vi "programacion practica de examen1.vi"() -> ()   [LabVIEW 2011]
panel:
  out "Array":T1(array[cluster]) {"diesel" scale=0.0..500.0; "Gasolina r" scale=0.0..500.0; "Gasolina S" scale=0.0..500.0}
  # "Existen 5 estaciones de servicio, ud debera de guardar las\nmediciones de los tanques de combustible de cada una de las\nestaciones de servicio y obtener el promedio mayor y menor\npor cada una de las estaciones y luego guardar los datos \nen un archivo de texto."
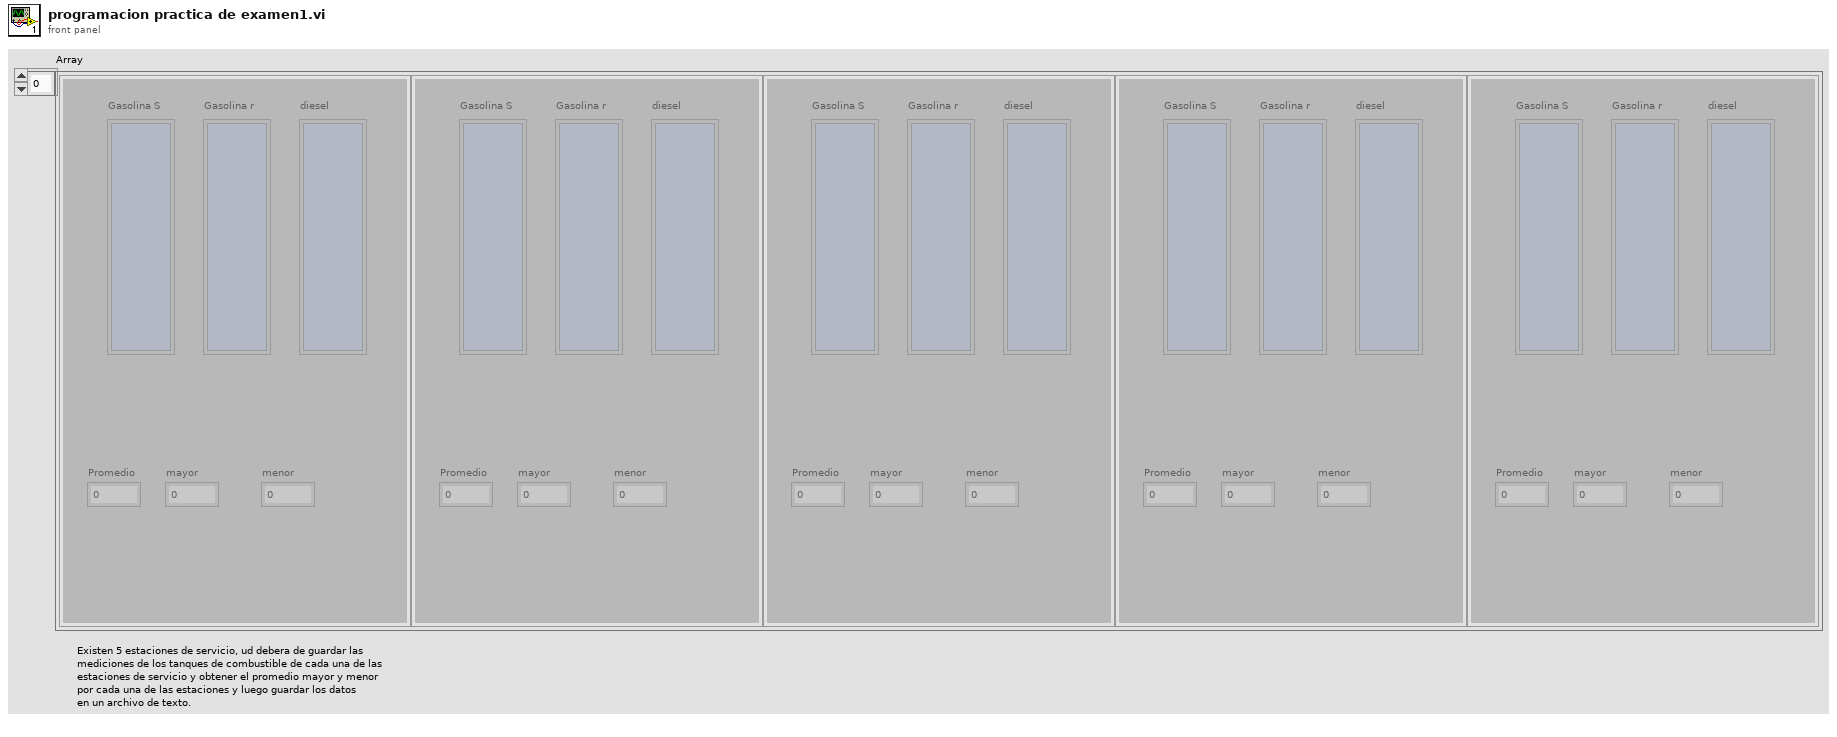
[diagram p1: front panel]
types:
  T1 = cluster{"Gasolina S":i32, "Gasolina r":i32, "diesel":i32, "Promedio":dbl, "mayor":dbl, "menor":dbl}[]
  T2 = enum16{"open", "replace", "create", "open or create", "replace or create", "replace or create with confirmation"}
  T3 = cluster{"Gasolina S":i32, "Gasolina r":i32, "diesel":i32, "Promedio":dbl, "mayor":dbl, "menor":dbl}
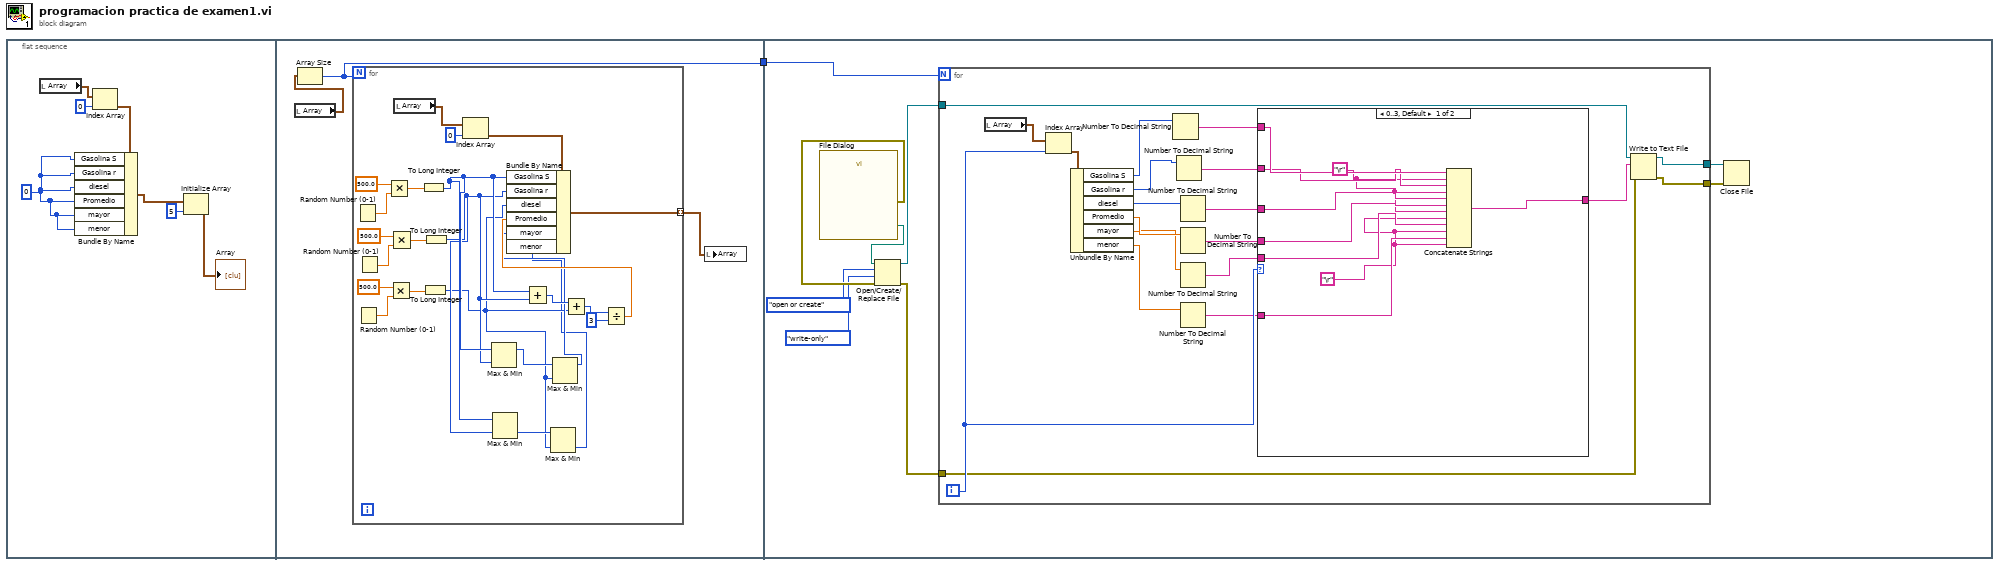
[diagram p0: block diagram]
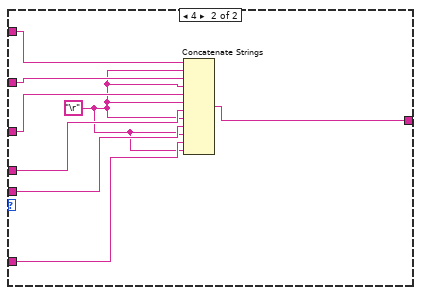
[diagram p2: hidden frame]
diagram:
  n1 = flat-sequence {
    tunnel: [w9] -> w1
    tunnel: w1 -> [w44]
    frame #0 {
      w5 = 0
      n2 = local read "Array"() -> (w8:T1)
      n3 = Index Array(array=w8, index=0) -> (element=w6:T3)
      n4 = Bundle By Name(cluster=w6, "Gasolina S"=w5, "Gasolina r"=w5, "diesel"=w5, "Promedio"=w5, "mayor"=w5, "menor"=w5) -> (w4:T3)
      n5 = Initialize Array(w4, 5 ("dimension size")) -> (→"Array":T1)
    }
    frame #1 {
      n6 = local read "Array"() -> (w11:T1)
      n7 = Array Size(array=w11) -> (size(s)=w9:i32)
      n8 = for {
        N: w9 -> [_]
        tunnel: [w12] -> w10 mode=indexing
        n9 = Random Number (0-1)() -> (number: 0 to 1=w31:dbl)
        n10 = Random Number (0-1)() -> (number: 0 to 1=w25:dbl)
        n11 = Random Number (0-1)() -> (number: 0 to 1=w28:dbl)
        n12 = Multiply(x=500.0, y=w31) -> (x*y=w30:dbl)
        n13 = Multiply(x=500.0, y=w25) -> (x*y=w24:dbl)
        n14 = Multiply(x=500.0, y=w28) -> (x*y=w29:dbl)
        n15 = local read "Array"() -> (w35:T1)
        n16 = To Long Integer(number=w30) -> (32bit integer=w17:i32)
        n17 = To Long Integer(number=w24) -> (32bit integer=w14:i32)
        n18 = To Long Integer(number=w29) -> (32bit integer=w16:i32)
        n19 = Index Array(array=w35, index=0) -> (element=w33:T3)
        n20 = Max & Min(x=w17, y=w16) -> (max(x,y)=w19:i32)  [unwired: 1 out]
        n21 = Max & Min(x=w17, y=w16) -> (min(x,y)=w15:i32)  [unwired: 1 out]
        n22 = Add(x=w17, y=w16) -> (x+y=w23:i32)
        n23 = Max & Min(x=w15, y=w14) -> (min(x,y)=w13:i32)  [unwired: 1 out]
        n24 = Max & Min(x=w19, y=w14) -> (max(x,y)=w18:i32)  [unwired: 1 out]
        n25 = Add(x=w23, y=w14) -> (x+y=w22:i32)
        n26 = Divide(x=w22, y=3) -> (x/y=w20:dbl)
        n27 = Bundle By Name(cluster=w33, "Gasolina S"=w17, "Gasolina r"=w16, "diesel"=w14, "Promedio"=w20, "mayor"=w18, "menor"=w13) -> (w12:T3)
      }
      n28 = local write "Array"(w10) -> ()
    }
    frame #2 {
      n29 = call "File Dialog"() -> ("selected path"=w43:path, "error out"=w42:errorcluster)  [unwired: 12 in, 2 out]
      n30 = Open/Create/Replace File(file path (use dialog)=w43, error in=w42, operation (0:open)=T2."open or create", access (0:read/write)=enum16{"read/write", "read-only", "write-only"}."write-only") -> (refnum out=w39:refnum<file>, error out=w38:errorcluster)  [unwired: 2 in, 1 out]
      n31 = for {
        N: w44 -> [_]
        tunnel: w39 -> [w48]
        tunnel: w38 -> [w47]
        tunnel: [w46] -> w37
        tunnel: [w45] -> w36
        i -> [w56]
        n32 = local read "Array"() -> (w64:T1)
        n33 = Index Array(array=w64, index=w56) -> (element=w63:T3)
        n34 = Unbundle By Name(w63) -> ("Gasolina S"=w62:i32, "Gasolina r"=w61:i32, "diesel"=w60:i32, "Promedio"=w59:dbl, "mayor"=w58:dbl, "menor"=w57:dbl)
        n35 = Number To Decimal String(number=w62) -> (decimal integer string=w55:string)  [unwired: 1 in]
        n36 = Number To Decimal String(number=w61) -> (decimal integer string=w54:string)  [unwired: 1 in]
        n37 = Number To Decimal String(number=w60) -> (decimal integer string=w53:string)  [unwired: 1 in]
        n38 = Number To Decimal String(number=w59) -> (decimal integer string=w52:string)  [unwired: 1 in]
        n39 = Number To Decimal String(number=w58) -> (decimal integer string=w51:string)  [unwired: 1 in]
        n40 = Number To Decimal String(number=w57) -> (decimal integer string=w50:string)  [unwired: 1 in]
        n41 = case shown="0..3, Default" w56 {
          tunnel: w55 -> [w72 w81]
          tunnel: w54 -> [w71 w80]
          tunnel: w53 -> [w70 w79]
          tunnel: w52 -> [w68 w78]
          tunnel: w51 -> [w67 w77]
          tunnel: w50 -> [w66 w76]
          tunnel: [w73 w74] -> w49
          frame 0..3, Default {
            w65 = "\r"
            w69 = "\r"
            n42 = Concatenate Strings(w72, w69, w71, w69, w70, w69, w68, w65, w67, w65, w66, w65) -> (w73:string)
          }
          frame 4 {
            w75 = "\r"
            n43 = Concatenate Strings(w81, w75, w80, w75, w79, w75, w78, w75, w77, w75, w76, w75) -> (w74:string)
          }
        }
        n44 = Write to Text File(file (use dialog)=w48, text=w49, error in=w47) -> (refnum out=w46:refnum<file>, error out=w45:errorcluster)  [unwired: 1 in, 1 out]
      }
      n45 = Close File(refnum=w37, error in=w36) -> ()  [unwired: 2 out]
    }
  }
